vi "Configuration Parse.vi"(8 "error in":errorcluster, 11 "UI Controls":T7={"measurement configuration"={"Automation Test"=FALSE, "Power sequencing file path"="", "RFmx name"="", "RFmx port"="", "DUT Max Gain (dB)"=0.0, "DUT Max Noise Figure (dB)"=0.0, "Reference Level Mode"=enum."Manual", "Reference Level (dBm)"=0.0, "Preamp Enabled"=0, "RFmx attenuation mode"=enum."<None>", "RFmx external attenuation (dB)"=0.0, "RFmx s-parameters orientation"=enum."Port1 Towards DUT", "RFmx s2p file path"="", "Switch Name"="", "Switch Connection"="", "ENS SMU Name"="", "ENS SMU Channel"="", "Action"=0, "Measurement Bandwidth (Hz)"=0.0, "Measurement Interval (s)"=0.0, "NF Cal Setup ID"="", "DUT Type"=0, "Frequency List Mode"=enum."Step", "Step - Start Frequency "=1000000000.0, "Step - Stop Frequency"=2000000000.0, "Step - Step Size"=100000000.0, "Points - Start Frequency"=1000000000.0, "Points - Stop Frequency"=2000000000.0, "Points - Number of Points"=11, "FreqList - Frequency List"=[], "Averaging Enabled"=FALSE, "Averaging Count"=0, "Noise Source Type"=0, "Noise Source RFSG Port"="port1", "Noise Source Cold Temperature (K)"=0.0, "Noise Source Off Temperature (K)"=0.0, "ENR Freq (Hz)"=[], "ENR (dB)"=[], "DUT Input_Compensation Enabled"=FALSE, "DUT Input_Temperation (K)"=0.0, "DUT Input_Loss Freq (Hz)"=[], "DUT Input_Loss (dB)"=[], "DUT Output_Compensation Enabled"=FALSE, "DUT Output_Temperation (K)"=0.0, "DUT Output_Loss Freq (Hz)"=[], "DUT Output_Loss (dB)"=[], "Calibration_Compensation Enabled"=FALSE, "Calibration_Temperation (K)"=0.0, "Calibration_Loss Freq (Hz)"=[], "Calibration_Loss (dB)"=[], "Noise Source_Compensation Enabled"=FALSE, "Noise Source_Temperation (K)"=0.0, "Noise Source_Loss Freq (Hz)"=[], "Noise Source_Loss (dB)"=[], "DUT Input Loss S2P File Path"="", "DUT Input Loss S-Parameter Orientation"=0, "DUT Output Loss S2P File Path"="", "DUT Output Loss S-Parameter Orientation"=0, "Calibration Loss S2P File Path"="", "Calibration Loss S-Parameter Orientation"=0, "Noise Source Loss S2P File Path"="", "Noise Source Loss S-Parameter Orientation"=0}, "measurement results"={"Status"="", "DUT NF vs Freq"=[], "Analyzer NF vs Freq"=[], "DUT NF (mean)"=0.0, "Analyzer NF (mean)"=0.0}} {"measurement configuration"."Noise Source Loss S-Parameter Orientation" items=["Port1 Towards DUT", "Port2 Towards DUT"]; "measurement configuration"."Calibration Loss S-Parameter Orientation" items=["Port1 Towards DUT", "Port2 Towards DUT"]; "measurement configuration"."DUT Output Loss S-Parameter Orientation" items=["Port1 Towards DUT", "Port2 Towards DUT"]; "measurement configuration"."DUT Input Loss S-Parameter Orientation" items=["Port1 Towards DUT", "Port2 Towards DUT"]; "measurement configuration"."FreqList - Frequency List" format="%.3p Hz"; "measurement configuration"."Points - Stop Frequency" format="%.3p Hz"; "measurement configuration"."Points - Start Frequency" format="%.3p Hz"; "measurement configuration"."Step - Step Size" format="%.3p Hz"; "measurement configuration"."Step - Stop Frequency" format="%.3p Hz"; "measurement configuration"."Step - Start Frequency" format="%.3p Hz"; "measurement configuration"."Noise Source_Loss (dB)" format="%.2g"; "measurement configuration"."Noise Source_Loss Freq (Hz)" format="%.3p"; "measurement configuration"."Noise Source_Temperation (K)" format="%.2g"; "measurement configuration"."Calibration_Loss (dB)" format="%.2g"; "measurement configuration"."Calibration_Loss Freq (Hz)" format="%.3p"; "measurement configuration"."Calibration_Temperation (K)" format="%.2g"; "measurement configuration"."DUT Output_Loss (dB)" format="%.2g"; "measurement configuration"."DUT Output_Loss Freq (Hz)" format="%.3p"; "measurement configuration"."DUT Output_Temperation (K)" format="%.2g"; "measurement configuration"."DUT Input_Loss (dB)" format="%.2g"; "measurement configuration"."DUT Input_Loss Freq (Hz)" format="%.3p"; "measurement configuration"."DUT Input_Temperation (K)" format="%.2g"; "measurement configuration"."ENR (dB)" format="%.2g"; "measurement configuration"."ENR Freq (Hz)" format="%.3p"; "measurement configuration"."Noise Source Off Temperature (K)" format="%.2f"; "measurement configuration"."Noise Source Cold Temperature (K)" format="%.2f"; "measurement configuration"."Noise Source Type" items=["External Noise Source", "RF Signal Generator"]; "measurement configuration"."DUT Type" items=["Amplifier", "Downconverter", "Upconverter"]; "measurement configuration"."Measurement Interval (s)" format="%.2p"; "measurement configuration"."Measurement Bandwidth (Hz)" format="%.3p"; "measurement configuration"."Action" items=["Measure", "Calibrate"]; "measurement configuration"."RFmx external attenuation (dB)" format="%.2f"; "measurement configuration"."Preamp Enabled" items=["Disabled"=0, "Enabled"=1, "Automatic"=3]; "measurement results"."Analyzer NF (mean)" format="%.2g"; "measurement results"."DUT NF (mean)" format="%.2g"; "measurement results"."Analyzer NF vs Freq" format="%.2g"; "measurement results"."DUT NF vs Freq" format="%.2g"}) -> (0 "error out":errorcluster, 1 "RFmx Settings":T8 {"Attenuation"."s2p File"."RFmx S-Parameters Orientation" items=["Port1 Towards DUT"=24000, "Port2 Towards DUT"=24001]; "Attenuation"."Constant Attenuation"."RFmx External Attenuation (dB)" format="%.2f"; "Preamp Enabled" items=["Disabled"=0, "Enabled"=1, "Automatic"=3]}, 3 "Test Configuration":T4={"Y-Factor Mode"=0, "Measurement Bandwidth (Hz)"=4000000.0, "Measurement Interval (s)"=0.1, "NF Cal Setup ID"="SNS_PS_6dB_ENR15_VI", "NF DUT Type"=0, "Frequency List (Hz)"=[4000000000.0, 9000000000.0], "Averaging"={"Enabled"=0, "Count"=10}, "Noise Source"={"Noise Source Type"=1, "Noise Source RFSG Port"="", "Cold Temperature (K)"=302.8, "Off Temperature (K)"=297.0, "ENR Freq (Hz)"=[6500000000.0], "ENR (dB)"=[15.0]}} {"Frequency List (Hz)" format="%.3p"; "NF DUT Type" items=["Amplifier", "Downconverter", "Upconverter"]; "Y-Factor Mode" items=["Measure", "Calibrate"]; "Noise Source"."Noise Source Type" items=["External Noise Source", "RF Signal Generator"]; "Noise Source"."ENR (dB)" format="%.2g"; "Noise Source"."ENR Freq (Hz)" format="%.3p"; "Noise Source"."Off Temperature (K)" format="%.2f"; "Noise Source"."Cold Temperature (K)" format="%.2f"; "Averaging"."Enabled" items=["False", "True"]; "Measurement Interval (s)" format="%.2p"; "Measurement Bandwidth (Hz)" format="%.3p"}, 4 "Switch":T1, 5 "Path Losses":T2={"DUT Input Loss"={"Compensation Enabled"=1, "Temperation (K)"=297.0, "S2P Path"=path "C:/Users/ies-pg-8881/Desktop/KB/CMT/PS_ATT6dB_26.5GHz.csv", "Orientation"=enum."Port1 Towards DUT"}, "DUT Output Loss"={"Compensation Enabled"=0, "Temperation (K)"=297.0, "S2P Path"=path "C:/Users/ies-pg-8881/Desktop/KB/CMT/PS_ATT6dB_26.5GHz.csv", "Orientation"=enum."Port1 Towards DUT"}, "Calibration Loss"={"Compensation Enabled"=1, "Temperation (K)"=297.0, "S2P Path"=path "C:/Users/ies-pg-8881/Desktop/KB/CMT/PS_ATT6dB_26.5GHz.csv", "Orientation"=enum."Port1 Towards DUT"}, "Noise Source Loss"={"Compensation Enabled"=0, "Temperation (K)"=297.0, "S2P Path"=path "C:/Users/ies-pg-8881/Desktop/KB/CMT/PS_ATT6dB_26.5GHz.csv", "Orientation"=enum."Port1 Towards DUT"}} {"Noise Source Loss"."Compensation Enabled" items=["False", "True"]; "Noise Source Loss"."Temperation (K)" format="%.2g"; "Calibration Loss"."Compensation Enabled" items=["False", "True"]; "Calibration Loss"."Temperation (K)" format="%.2g"; "DUT Output Loss"."Compensation Enabled" items=["False", "True"]; "DUT Output Loss"."Temperation (K)" format="%.2g"; "DUT Input Loss"."Compensation Enabled" items=["False", "True"]; "DUT Input Loss"."Temperation (K)" format="%.2g"})   [LabVIEW 2023, in "FPT NoiseFigure.lvclass"]
uses:
  FPT NoiseFigure.lvclass
  Measurement/Controls/RFmx Config - NF.ctl
  Measurement Configuration.ctl
  Measurement Results.ctl
  Measurement/Controls/Test Config - NF.ctl
  Measurement/Controls/Path Loss Settings Cluster.ctl
  Measurement/Controls/Path Loss Settings.ctl
  Measurement/Controls/Switches - NF.ctl
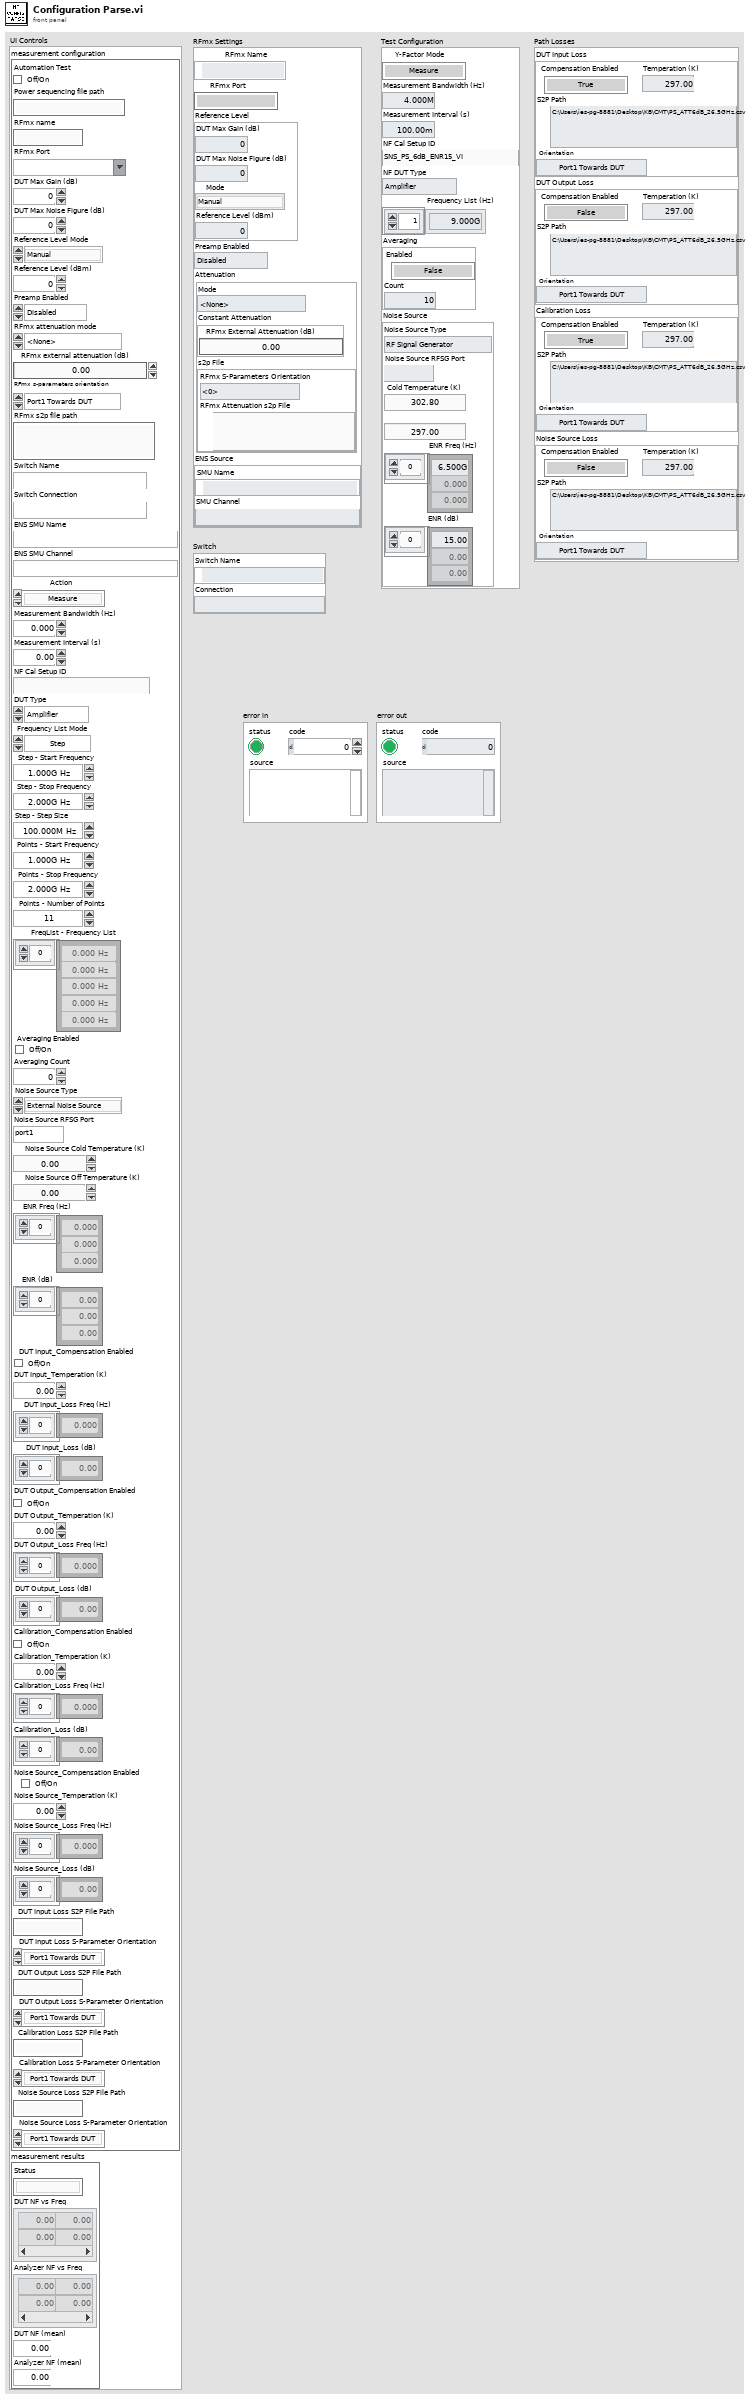
[diagram p1: front panel]
types:
  T1 = typedef "Switches - NF.ctl" = cluster{"Switch Name":refnum<k15>, "Connection":string}
  T2 = typedef "Path Loss Settings Cluster.ctl" = cluster{"DUT Input Loss":T3, "DUT Output Loss":T3, "Calibration Loss":T3, "Noise Source Loss":T3}
  T3 = typedef "Path Loss Settings.ctl" = cluster{"Compensation Enabled":i32, "Temperation (K)":dbl, "S2P Path":path, "Orientation":enum32{"Port1 Towards DUT", "Port2 Towards DUT"}}
  T4 = typedef "Test Config - NF.ctl" = cluster{"Y-Factor Mode":i32, "Measurement Bandwidth (Hz)":dbl, "Measurement Interval (s)":dbl, "NF Cal Setup ID":string, "NF DUT Type":i32, "Frequency List (Hz)":dbl[], "Averaging":cluster{"Enabled":i32, "Count":i32}, "Noise Source":cluster{"Noise Source Type":i32, "Noise Source RFSG Port":string, "Cold Temperature (K)":dbl, "Off Temperature (K)":dbl, "ENR Freq (Hz)":dbl[], "ENR (dB)":dbl[]}}
  T5 = typedef "FPT NoiseFigure.lvclass/Measurement Configuration.ctl" = cluster{"Automation Test":bool, "Power sequencing file path":string, "RFmx name":string, "RFmx port":string, "DUT Max Gain (dB)":dbl, "DUT Max Noise Figure (dB)":dbl, "Reference Level Mode":enum32{"Manual", "Recommend"}, "Reference Level (dBm)":dbl, "Preamp Enabled":i32, "RFmx attenuation mode":enum32{"<None>", "Constant Attenuation", "s2p File"}, "RFmx external attenuation (dB)":dbl, "RFmx s-parameters orientation":enum32{"Port1 Towards DUT", "Port2 Towards DUT"}, "RFmx s2p file path":string, "Switch Name":string, "Switch Connection":string, "ENS SMU Name":string, "ENS SMU Channel":string, "Action":u32, "Measurement Bandwidth (Hz)":dbl, "Measurement Interval (s)":dbl, "NF Cal Setup ID":string, "DUT Type":i32, "Frequency List Mode":enum32{"Step", "Points", "Frequency List"}, "Step - Start Frequency ":dbl, "Step - Stop Frequency":dbl, "Step - Step Size":dbl, "Points - Start Frequency":dbl, "Points - Stop Frequency":dbl, "Points - Number of Points":i32, "FreqList - Frequency List":dbl[], "Averaging Enabled":bool, "Averaging Count":i32, "Noise Source Type":i32, "Noise Source RFSG Port":string, "Noise Source Cold Temperature (K)":dbl, "Noise Source Off Temperature (K)":dbl, "ENR Freq (Hz)":dbl[], "ENR (dB)":dbl[], "DUT Input_Compensation Enabled":bool, "DUT Input_Temperation (K)":dbl, "DUT Input_Loss Freq (Hz)":dbl[], "DUT Input_Loss (dB)":dbl[], "DUT Output_Compensation Enabled":bool, "DUT Output_Temperation (K)":dbl, "DUT Output_Loss Freq (Hz)":dbl[], "DUT Output_Loss (dB)":dbl[], "Calibration_Compensation Enabled":bool, "Calibration_Temperation (K)":dbl, "Calibration_Loss Freq (Hz)":dbl[], "Calibration_Loss (dB)":dbl[], "Noise Source_Compensation Enabled":bool, "Noise Source_Temperation (K)":dbl, "Noise Source_Loss Freq (Hz)":dbl[], "Noise Source_Loss (dB)":dbl[], "DUT Input Loss S2P File Path":string, "DUT Input Loss S-Parameter Orientation":i32, "DUT Output Loss S2P File Path":string, "DUT Output Loss S-Parameter Orientation":i32, "Calibration Loss S2P File Path":string, "Calibration Loss S-Parameter Orientation":i32, "Noise Source Loss S2P File Path":string, "Noise Source Loss S-Parameter Orientation":i32}
  T6 = typedef "FPT NoiseFigure.lvclass/Measurement Results.ctl" = cluster{"Status":string, "DUT NF vs Freq":dbl[][], "Analyzer NF vs Freq":dbl[][], "DUT NF (mean)":dbl, "Analyzer NF (mean)":dbl}
  T7 = cluster{"measurement configuration":T5, "measurement results":T6}
  T8 = typedef "RFmx Config - NF.ctl" = cluster{"RFmx Name":refnum<k15>, "RFmx Port":string, "Reference Level":cluster{"DUT Max Gain (dB)":dbl, "DUT Max Noise Figure (dB)":dbl, "Mode":enum32{"Manual", "Recommend"}, "Reference Level (dBm)":dbl}, "Preamp Enabled":i32, "Attenuation":cluster{"Mode":enum32{"<None>", "Constant Attenuation", "s2p File"}, "Constant Attenuation":cluster{"RFmx External Attenuation (dB)":dbl}, "s2p File":cluster{"RFmx S-Parameters Orientation":i32, "RFmx Attenuation s2p File":path}}, "ENS Source":cluster{"SMU Name":refnum<k15>, "SMU Channel":string}}
  T9 = enum32{"<None>", "Constant Attenuation", "s2p File"}
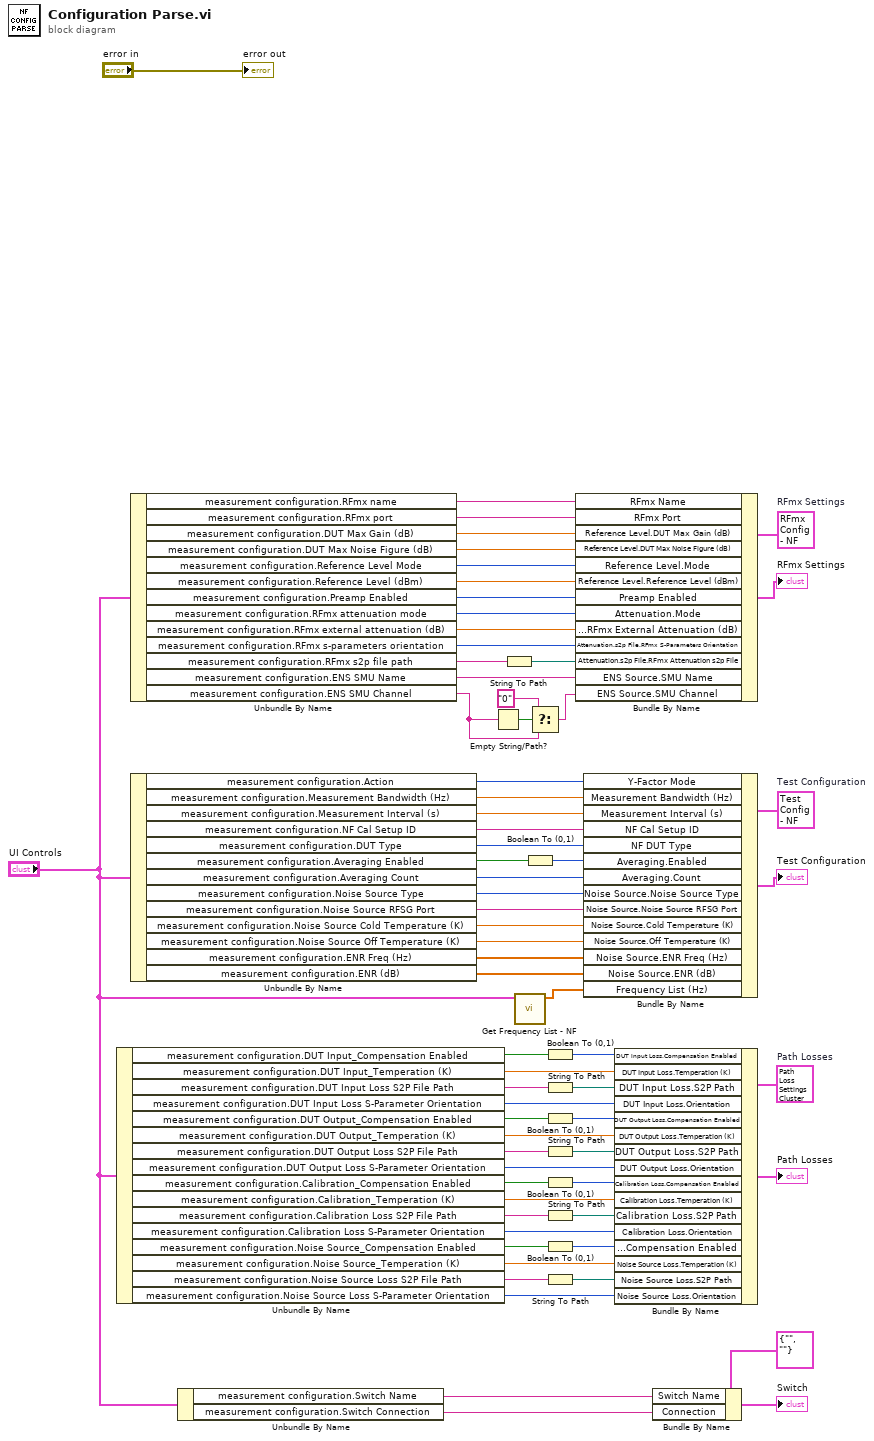
[diagram p0: block diagram]
diagram:
  w41 = T2 {"DUT Input Loss"={"Compensation Enabled"=1, "Temperation (K)"=297.0, "S2P Path"=path "C:/Users/ies-pg-8881/Desktop/KB/CMT/PS_ATT6dB_26.5GHz.csv", "Orientation"=enum."Port1 Towards DUT"}, "DUT Output Loss"={"Compensation Enabled"=0, "Temperation (K)"=297.0, "S2P Path"=path "C:/Users/ies-pg-8881/Desktop/KB/CMT/PS_ATT6dB_26.5GHz.csv", "Orientation"=enum."Port1 Towards DUT"}, "Calibration Loss"={"Compensation Enabled"=1, "Temperation (K)"=297.0, "S2P Path"=path "C:/Users/ies-pg-8881/Desktop/KB/CMT/PS_ATT6dB_26.5GHz.csv", "Orientation"=enum."Port1 Towards DUT"}, "Noise Source Loss"={"Compensation Enabled"=0, "Temperation (K)"=297.0, "S2P Path"=path "C:/Users/ies-pg-8881/Desktop/KB/CMT/PS_ATT6dB_26.5GHz.csv", "Orientation"=enum."Port1 Towards DUT"}}  # Path Losses
  w54 = T4 {"Y-Factor Mode"=0, "Measurement Bandwidth (Hz)"=4000000.0, "Measurement Interval (s)"=0.1, "NF Cal Setup ID"="SNS_PS_6dB_ENR15_26.5GHz_VI", "NF DUT Type"=0, "Frequency List (Hz)"=[4000000000.0, 5000000000.0, 6000000000.0, 7000000000.0, 8000000000.0, 9000000000.0, 10000000000.0, 11000000000.0, 12000000000.0, 13000000000.0, 14000000000.0, 15000000000.0, 16000000000.0, 17000000000.0, 18000000000.0, 19000000000.0, 20000000000.0], "Averaging"={"Enabled"=0, "Count"=10}, "Noise Source"={"Noise Source Type"=1, "Noise Source RFSG Port"="", "Cold Temperature (K)"=302.8, "Off Temperature (K)"=297.0, "ENR Freq (Hz)"=[6500000000.0], "ENR (dB)"=[15.0]}}  # Test Configuration
  w56 = T8 {"RFmx Name"="5842_0", "RFmx Port"="", "Reference Level"={"DUT Max Gain (dB)"=17.5, "DUT Max Noise Figure (dB)"=3.0, "Mode"=enum."Recommend", "Reference Level (dBm)"=0.0}, "Preamp Enabled"=3, "Attenuation"={"Mode"=enum."Constant Attenuation", "Constant Attenuation"={"RFmx External Attenuation (dB)"=0.8}, "s2p File"={"RFmx S-Parameters Orientation"=24000, "RFmx Attenuation s2p File"=path ""}}, "ENS Source"={"SMU Name"="", "SMU Channel"=""}}  # RFmx Settings
  n1 = Unbundle By Name("UI Controls") -> ("measurement configuration.DUT Input_Compensation Enabled"=w40:bool, "measurement configuration.DUT Input_Temperation (K)"=w39:dbl, "measurement configuration.DUT Input Loss S2P File Path"=w38:string, "measurement configuration.DUT Input Loss S-Parameter Orientation"=w37:i32, "measurement configuration.DUT Output_Compensation Enabled"=w36:bool, "measurement configuration.DUT Output_Temperation (K)"=w35:dbl, "measurement configuration.DUT Output Loss S2P File Path"=w34:string, "measurement configuration.DUT Output Loss S-Parameter Orientation"=w33:i32, "measurement configuration.Calibration_Compensation Enabled"=w32:bool, "measurement configuration.Calibration_Temperation (K)"=w31:dbl, "measurement configuration.Calibration Loss S2P File Path"=w30:string, "measurement configuration.Calibration Loss S-Parameter Orientation"=w29:i32, "measurement configuration.Noise Source_Compensation Enabled"=w28:bool, "measurement configuration.Noise Source_Temperation (K)"=w27:dbl, "measurement configuration.Noise Source Loss S2P File Path"=w26:string, "measurement configuration.Noise Source Loss S-Parameter Orientation"=w25:i32)
  n2 = Unbundle By Name("UI Controls") -> ("measurement configuration.RFmx name"=w68:string, "measurement configuration.RFmx port"=w67:string, "measurement configuration.DUT Max Gain (dB)"=w66:dbl, "measurement configuration.DUT Max Noise Figure (dB)"=w65:dbl, "measurement configuration.Reference Level Mode"=w64:enum32{"Manual", "Recommend"}, "measurement configuration.Reference Level (dBm)"=w63:dbl, "measurement configuration.Preamp Enabled"=w62:i32, "measurement configuration.RFmx attenuation mode"=w61:T9, "measurement configuration.RFmx external attenuation (dB)"=w60:dbl, "measurement configuration.RFmx s-parameters orientation"=w59:enum32{"Port1 Towards DUT", "Port2 Towards DUT"}, "measurement configuration.RFmx s2p file path"=w58:string, "measurement configuration.ENS SMU Name"=w12:string, "measurement configuration.ENS SMU Channel"=w10:string)
  n3 = Unbundle By Name("UI Controls") -> ("measurement configuration.Action"=w53:u32, "measurement configuration.Measurement Bandwidth (Hz)"=w52:dbl, "measurement configuration.Measurement Interval (s)"=w51:dbl, "measurement configuration.NF Cal Setup ID"=w50:string, "measurement configuration.DUT Type"=w49:i32, "measurement configuration.Averaging Enabled"=w48:bool, "measurement configuration.Averaging Count"=w47:i32, "measurement configuration.Noise Source Type"=w46:i32, "measurement configuration.Noise Source RFSG Port"=w6:string, "measurement configuration.Noise Source Cold Temperature (K)"=w7:dbl, "measurement configuration.Noise Source Off Temperature (K)"=w45:dbl, "measurement configuration.ENR Freq (Hz)"=w44:dbl[], "measurement configuration.ENR (dB)"=w43:dbl[])
  n4 = Unbundle By Name("UI Controls") -> ("measurement configuration.Switch Name"=w3:string, "measurement configuration.Switch Connection"=w2:string)
  n5 = Empty String/Path?(string/path=w10) -> (empty?=w11:bool)
  n6 = String To Path(string=w58) -> (path=w57:path)
  n7 = call "Get Frequency List - NF.vi"("UI Controls"="UI Controls") -> ("Frequency List"=w22:dbl[])  [unwired: 10 in]
  n8 = Boolean To (0,1)(Boolean=w48) -> (0, 1=w21:i16)
  n9 = Select(t="0", s=w11, f=w10) -> (s? t:f=w9:string)
  n10 = Boolean To (0,1)(Boolean=w40) -> (0, 1=w20:i16)
  n11 = String To Path(string=w38) -> (path=w16:path)
  n12 = Boolean To (0,1)(Boolean=w36) -> (0, 1=w19:i16)
  n13 = String To Path(string=w34) -> (path=w15:path)
  n14 = Boolean To (0,1)(Boolean=w32) -> (0, 1=w18:i16)
  n15 = String To Path(string=w30) -> (path=w14:path)
  n16 = Boolean To (0,1)(Boolean=w28) -> (0, 1=w17:i16)
  n17 = String To Path(string=w26) -> (path=w13:path)
  n18 = Bundle By Name(cluster=w56, "RFmx Name"=w68, "RFmx Port"=w67, "Reference Level.DUT Max Gain (dB)"=w66, "Reference Level.DUT Max Noise Figure (dB)"=w65, "Reference Level.Mode"=w64, "Reference Level.Reference Level (dBm)"=w63, "Preamp Enabled"=w62, "Attenuation.Mode"=w61, "Attenuation.Constant Attenuation.RFmx External Attenuation (dB)"=w60, "Attenuation.s2p File.RFmx S-Parameters Orientation"=w59, "Attenuation.s2p File.RFmx Attenuation s2p File"=w57, "ENS Source.SMU Name"=w12, "ENS Source.SMU Channel"=w9) -> (→"RFmx Settings":T8)
  n19 = Bundle By Name(cluster=w54, "Y-Factor Mode"=w53, "Measurement Bandwidth (Hz)"=w52, "Measurement Interval (s)"=w51, "NF Cal Setup ID"=w50, "NF DUT Type"=w49, "Averaging.Enabled"=w21, "Averaging.Count"=w47, "Noise Source.Noise Source Type"=w46, "Noise Source.Noise Source RFSG Port"=w6, "Noise Source.Cold Temperature (K)"=w7, "Noise Source.Off Temperature (K)"=w45, "Noise Source.ENR Freq (Hz)"=w44, "Noise Source.ENR (dB)"=w43, "Frequency List (Hz)"=w22) -> (→"Test Configuration":T4)
  n20 = Bundle By Name(cluster=w41, "DUT Input Loss.Compensation Enabled"=w20, "DUT Input Loss.Temperation (K)"=w39, "DUT Input Loss.S2P Path"=w16, "DUT Input Loss.Orientation"=w37, "DUT Output Loss.Compensation Enabled"=w19, "DUT Output Loss.Temperation (K)"=w35, "DUT Output Loss.S2P Path"=w15, "DUT Output Loss.Orientation"=w33, "Calibration Loss.Compensation Enabled"=w18, "Calibration Loss.Temperation (K)"=w31, "Calibration Loss.S2P Path"=w14, "Calibration Loss.Orientation"=w29, "Noise Source Loss.Compensation Enabled"=w17, "Noise Source Loss.Temperation (K)"=w27, "Noise Source Loss.S2P Path"=w13, "Noise Source Loss.Orientation"=w25) -> (→"Path Losses":T2)
  n21 = Bundle By Name(cluster=T1 {"Switch Name"="", "Connection"=""} ("Switch"), "Switch Name"=w3, "Connection"=w2) -> (→"Switch":T1)
  "error out" <- "error in"
